vi "keithley_init.vi"(7 "Output Level (0)":dbl, 8 "error in (no error)":errorcluster, 9 "Compliance  Level (0.1)":dbl=2.1, 10 "Source Mode  (0: Voltage)":u16(ring)=1 items=["Voltage", "Current"], 11 "VISA resource name":refnum<visa-resource-name>) -> (0 "error out":errorcluster, 3 "VISA resource name out":refnum<visa-resource-name>)   [LabVIEW 2023]
uses:
  keithley_24xx/Keithley 24XX/Keithley 24XX.lvlib
panel:
  in  "Output Off Behavior (0: Normal)":u16(ring)=1 items=["Normal", "High Impedance", "Zero", "Guard"]
  in  "Displayed Measurement (0: Voltage)":u16(ring) items=["Voltage", "Current", "Resistance"]
  in  "Enable Voltage Auto Range (T:Enable)":bool=TRUE
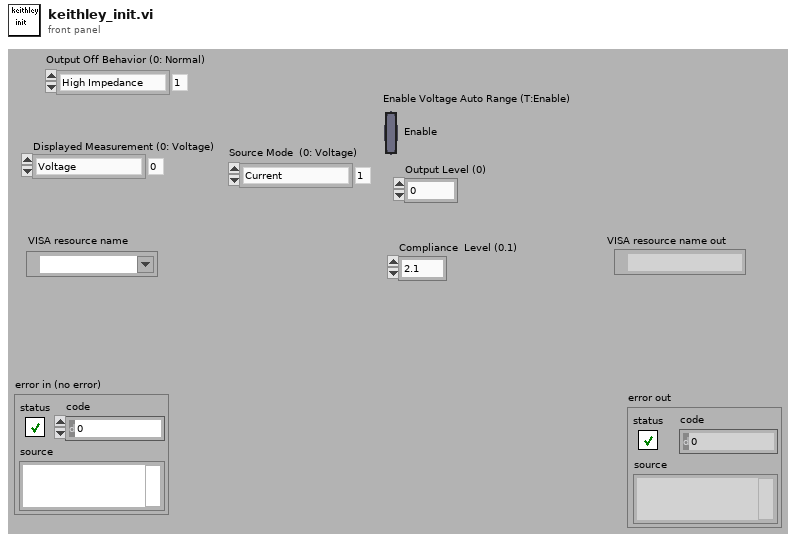
[diagram p1: front panel]
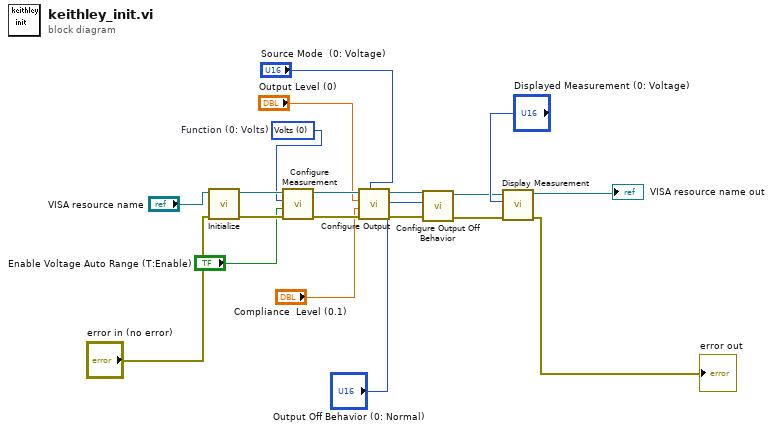
[diagram p0: block diagram]
diagram:
  w15 = u16 0 items=["Volts", "Current", "Resistance"]  # Function (0: Volts)
  n1 = call "Initialize.vi"("error in (no error)"="error in (no error)", "VISA resource name"="VISA resource name") -> ("error out"=w16:errorcluster, "VISA resource name out"=w17:refnum<visa-resource-name>)  [unwired: 8 in]
  n2 = call "Configure Measurement.vi"("error in (no error)"=w16, "Enable Auto Range (T:Enable)"="Enable Voltage Auto Range (T:Enable)", "Function (0: Volts)"=w15, "VISA resource name"=w17) -> ("error out"=w12:errorcluster, "VISA resource name out"=w13:refnum<visa-resource-name>)  [unwired: 6 in]
  n3 = call "Configure Output.vi"("Source Mode  (0: Voltage)"="Source Mode  (0: Voltage)", "error in (no error)"=w12, "Compliance  Level (0.1)"="Compliance  Level (0.1)", "Output Level (0)"="Output Level (0)", "VISA resource name"=w13) -> ("error out"=w3:errorcluster, "VISA resource name out"=w4:refnum<visa-resource-name>)  [unwired: 5 in]
  n4 = call "Configure Output Off Behavior.vi"("error in (no error)"=w3, "Output Off Behavior (0: Normal)"="Output Off Behavior (0: Normal)", "VISA resource name"=w4) -> ("error out"=w1:errorcluster, "VISA resource name out"=w2:refnum<visa-resource-name>)  [unwired: 7 in]
  n5 = call "Display Measurement.vi"("error in (no error)"=w1, "Displayed Measurement (0: Voltage)"="Displayed Measurement (0: Voltage)", "VISA resource name"=w2) -> ("error out"=→"error out":errorcluster, "VISA resource name out"=→"VISA resource name out":refnum<visa-resource-name>)  [unwired: 7 in]
